vi "Set Iteration.vi"(7 "Progress Max":i32, 8 "error in (no error)":errorcluster {"code" format="Error %.0f"}, 9 "Progress Value":i32, 10 "Message (No Message Update)":string, 11 "VIDoc Printer In":refnum<class "VIDoc Printer.lvclass">) -> (0 "error out":errorcluster {"code" format="Error %.0f"}, 2 "Abort?":bool, 3 "VIDoc Printer Out":refnum<class "VIDoc Printer.lvclass">)   [LabVIEW 2023, in "VIDoc Printer.lvlib" / "VIDoc Printer.lvclass"]
uses:
  VIDoc Printer.lvclass
  VIDoc Printer.lvclass/VIDoc Printer.ctl
  UI Interaction/UI Interaction.lvclass
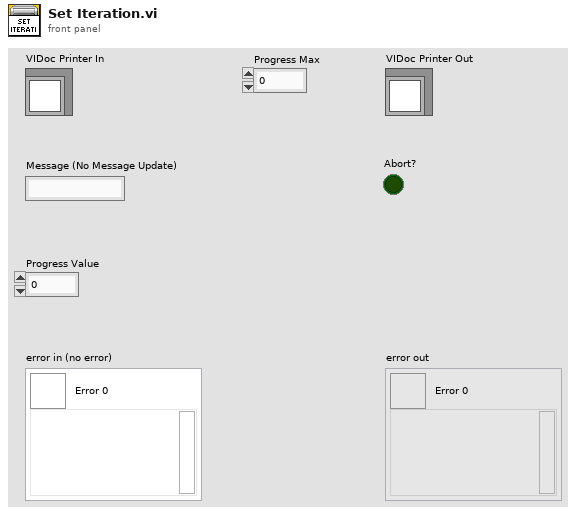
[diagram p1: front panel]
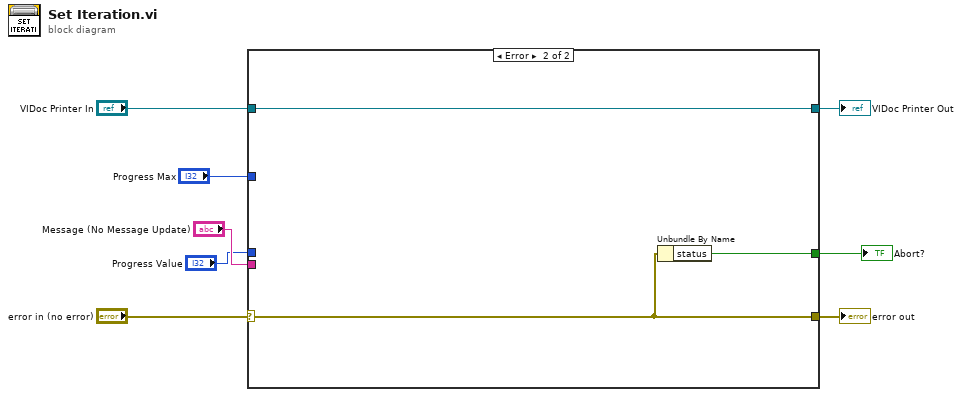
[diagram p0: block diagram]
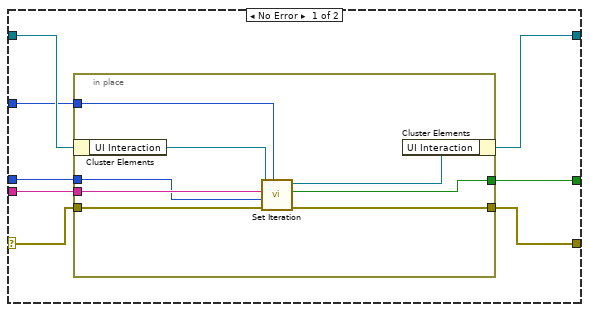
[diagram p2: hidden frame]
diagram:
  n1 = case shown="Error" "error in (no error)" {
    selector: "error in (no error)" -> [w14 w26]
    tunnel: [w13 w26] -> w7
    tunnel: [w16 w27] -> w5
    tunnel: "VIDoc Printer In" -> [w15 w27]
    tunnel: "Progress Max" -> [w12 _]
    tunnel: "Message (No Message Update)" -> [w11 _]
    tunnel: "Progress Value" -> [w10 _]
    tunnel: [w9 w25] -> w1
    frame No Error {
      n2 = in-place {
        in-place-border: w14 -> [w22]
        in-place-border: [w21] -> w13
        in-place-border: w12 -> [w20]
        in-place-border: w11 -> [w19]
        in-place-border: w10 -> [w18]
        in-place-border: [w17] -> w9
        n3 = in-place-cluster #1(w15) -> ("UI Interaction"=w24:refnum<class "UI Interaction.lvclass">)
        n4 = call "Set Iteration.vi"("Progress Max"=w20, "error in (no error)"=w22, "Progress Value"=w18, "Message (No Message Update)"=w19, "UI Interaction in"=w24) -> ("error out"=w21:errorcluster, "Abort?"=w17:bool, "UI Interaction out"=w23:refnum<class "UI Interaction.lvclass">)  [unwired: 4 in]
        n5 = in-place-cluster #1("UI Interaction"=w23) -> (w16:refnum<class "VIDoc Printer.lvclass">)
      }
    }
    frame Error {
      n6 = Unbundle By Name(w26) -> ("status"=w25:bool)
    }
  }
  "error out" <- w7
  "VIDoc Printer Out" <- w5
  "Abort?" <- w1
